vi "Get DVR.vi"(0 "Class Path":path, 11 "Error in":errorcluster) -> (4 "Device DVR":refnum<data-value>, 15 "Error out":errorcluster)   [LabVIEW 2020, in "Device.lvclass"]
doc: "Get class object from the path and generates DVR for the class object."
uses:
  Device.lvclass
panel:
  out "Device out":refnum<class "Device.lvclass">
  in  "Device in":refnum<class "Device.lvclass">
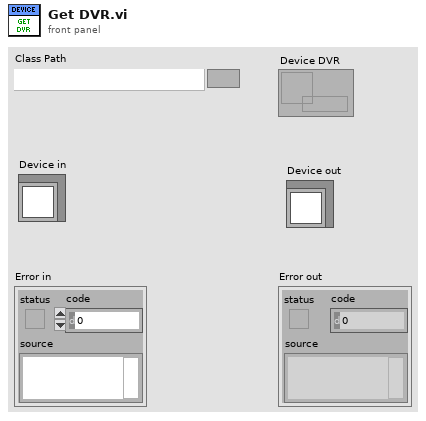
[diagram p1: front panel]
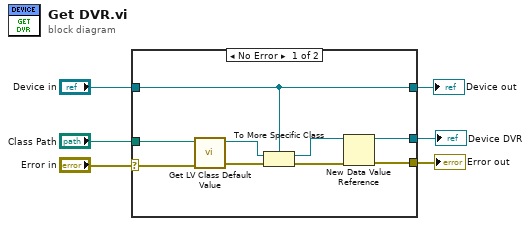
[diagram p0: block diagram]
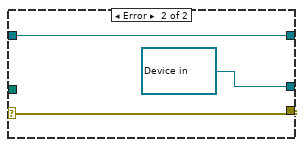
[diagram p2: hidden frame]
diagram:
  n1 = case shown="No Error" "Error in" {
    selector: "Error in" -> [w15 w18]
    tunnel: [w7 w18] -> w5
    tunnel: [w11 w17] -> w3
    tunnel: "Device in" -> [w11 w17]
    tunnel: "Class Path" -> [w14 _]
    tunnel: [w8 refnum<data-value> refnum ("data value reference")] -> w1
    frame No Error {
      n2 = call <vilib>:"Get LV Class Default Value.vi"("error in (no error)"=w15, "class path"=w14) -> ("error out"=w13:errorcluster, "object"=w12:refnum<class>)  [unwired: 8 in]
      n3 = To More Specific Class(target class=w11, reference=w12, error in=w13) -> (specific class reference=w9:refnum<class "Device.lvclass">, error out=w10:errorcluster)
      n4 = New Data Value Reference(data value=w9, error in=w10) -> (data value reference=w8:refnum<data-value>, error out=w7:errorcluster)
    }
    frame Error {
    }
  }
  "Error out" <- w5
  "Device out" <- w3
  "Device DVR" <- w1
